vi "传感器参数读取.vi"(8 "Error in":errorcluster caption="Error in (no error)") -> (0 "error out":errorcluster, 3 "添加的数组":string[][](array[string]))   [LabVIEW 2016, in "斯坦道仪器.lvlib"]
panel:
  in  "传感器区":i32(listbox)
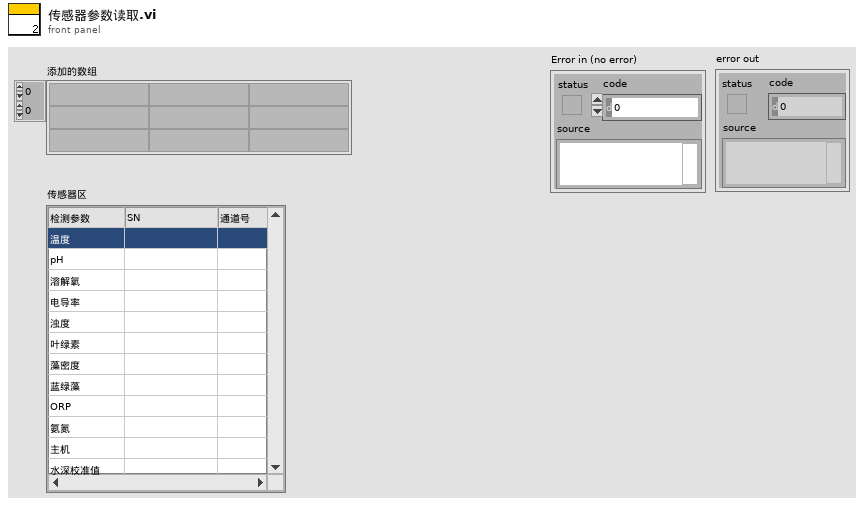
[diagram p1: front panel]
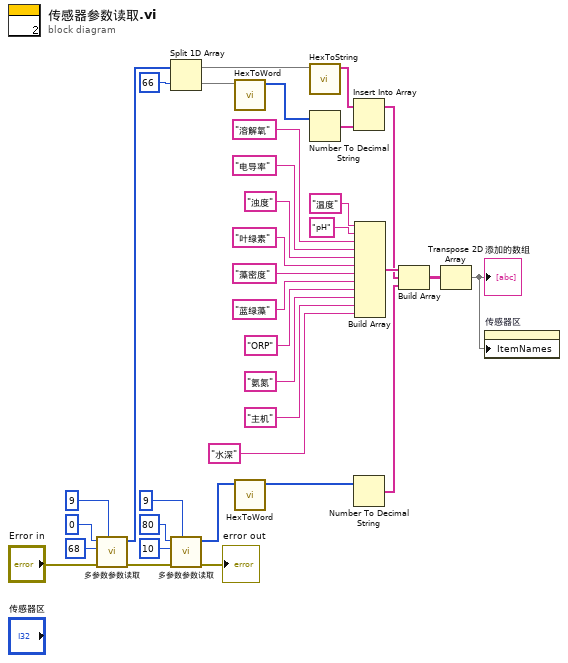
[diagram p0: block diagram]
diagram:
  n1 = call "多参数参数读取.vi"("Slave ID"=u8 9, "Error in"="Error in", "quantity"=u16 68, "starting address"=u16 0) -> ("error out"=w32:errorcluster, "Registers"=w28:u16[])  [unwired: 6 in]
  n2 = Split 1D Array(array=w28, index=66 ("索引")) -> (first subarray=w26:u16[], second subarray=w25:u16[])
  n3 = call "多参数参数读取.vi"("Slave ID"=u8 9, "Error in"=w32, "quantity"=u16 10, "starting address"=u16 80) -> ("error out"=→"error out":errorcluster, "Registers"=w2:u16[])  [unwired: 6 in]
  n4 = call "HexToWord.vi"("数组"=w25) -> ("WORD"=w11:u16[])  [unwired: 10 in]
  n5 = call "HexToWord.vi"("数组"=w2) -> ("WORD"=w1:u16[])  [unwired: 10 in]
  n6 = call "HexToString.vi"("数组"=w26) -> ("STRING"=w12:string[])  [unwired: 10 in]
  n7 = Number To Decimal String(number=w11) -> (decimal integer string=w10:string[])  [unwired: 1 in]
  n8 = Insert Into Array(array=w12, new element=w10) -> (w8:string[])  [unwired: 1 in]
  n9 = Number To Decimal String(number=w1) -> (decimal integer string=w7:string[])  [unwired: 1 in]
  n10 = Build Array("温度", "pH", "溶解氧", "电导率", "浊度", "叶绿素", "藻密度", "蓝绿藻", "ORP", "氨氮", "主机", "水深") -> (w9:string[])
  n11 = Build Array(w9, w8, w7) -> (w6:string[][])
  n12 = Transpose 2D Array(2D array=w6) -> (transposed array=w5:string[][])
  "添加的数组" <- w5
  n13 = property on="传感器区" class="MCListbox (严格)"("ItemNames"=w5) -> ()  [unwired: 2 in, 2 out]
